vi "MIO Get QCurve Multi.vi"(1 "Lower Limit":sgl format="%.2f", 2 "Upper Limit":sgl format="%.2f", 3 "Num Sweeps":i32=1) -> (0 "Waveform Graph":dbl[](graph))   [LabVIEW 2009]
uses:
  <vilib>/Daq/zadvd.llb/AO Buffer Write (scaled array).vi
  QCA Global.vi
  <vilib>/Daq/Ai.llb/AI Read (scaled array).vi
panel:
  in  "Multiplicity":i32=1
  out "Tune":dbl(slide) scale=-1.0..1.0 scale format="%.2f"
  out "Triangle Wave":dbl[](graph)=[-1.0, -0.996, -0.992, -0.988, -0.984, -0.98, -0.976, -0.972, -0.968, -0.964, -0.96, -0.956, -0.952, -0.948, -0.944, -0.94, -0.9359999999999999, -0.9319999999999999, -0.928, -0.924, -0.92, -0.916, -0.912, -0.908, -0.904, -0.9, -0.896, -0.892, -0.888, -0.884, -0.88, -0.876, -0.872, -0.868, -0.864, -0.86, -0.856, -0.852, -0.848, -0.844, -0.84, -0.836, -0.832, -0.8280000000000001, -0.8240000000000001, -0.8200000000000001, -0.8160000000000001, -0.812, -0.808, -0.804, -0.8, -0.796, -0.792, -0.788, -0.784, -0.78, -0.776, -0.772, -0.768, -0.764, -0.76, -0.756, -0.752, -0.748, -0.744, -0.74, -0.736, -0.732, -0.728, -0.724, -0.72, -0.716, -0.712, -0.708, -0.704, -0.7, -0.696, -0.692, -0.688, -0.6839999999999999, -0.6799999999999999, -0.6759999999999999, -0.6719999999999999, -0.6679999999999999, -0.6639999999999999, -0.6599999999999999, -0.656, -0.652, -0.648, -0.644, -0.64, -0.636, -0.632, -0.628, -0.624, -0.62, -0.616, -0.612, -0.608, -0.604, -0.6, -0.596, -0.5920000000000001, -0.5880000000000001, -0.5840000000000001, -0.5800000000000001, -0.5760000000000001, -0.5720000000000001, -0.5680000000000001, -0.5640000000000001, -0.56, -0.556, -0.552, -0.548, -0.544, -0.54, -0.536, -0.532, -0.528, -0.524, -0.52, -0.516, -0.512, -0.508, -0.504, -0.5, -0.496, -0.492, -0.488, -0.484, -0.48, -0.476, -0.472, -0.46799999999999997, -0.46399999999999997, -0.45999999999999996, -0.45599999999999996, -0.45199999999999996, -0.44799999999999995, -0.44399999999999995, -0.43999999999999995, -0.43600000000000005, -0.43200000000000005, -0.42800000000000005, -0.42400000000000004, -0.42000000000000004, -0.41600000000000004, -0.41200000000000003, -0.40800000000000003, -0.404, -0.4, -0.396, -0.392, -0.388, -0.384, -0.38, -0.376, -0.372, -0.368, -0.364, -0.36, -0.356, -0.352, -0.348, -0.344, -0.33999999999999997, -0.33599999999999997, -0.33199999999999996, -0.32799999999999996, -0.32399999999999995, -0.31999999999999995, -0.31599999999999995, -0.31200000000000006, -0.30800000000000005, -0.30400000000000005, -0.30000000000000004, -0.29600000000000004, -0.29200000000000004, -0.28800000000000003, -0.28400000000000003, -0.28, -0.276, -0.272, -0.268, -0.264, -0.26, -0.256, -0.252, -0.248, -0.244, -0.24, -0.236, -0.23199999999999998, -0.22799999999999998, -0.22399999999999998, -0.21999999999999997, -0.21599999999999997, -0.21199999999999997, -0.20799999999999996, -0.20399999999999996, -0.19999999999999996, -0.19599999999999995, -0.19199999999999995, -0.18799999999999994, -0.18400000000000005, -0.18000000000000005, -0.17600000000000005, -0.17200000000000004, -0.16800000000000004, -0.16400000000000003, -0.16000000000000003, -0.15600000000000003, -0.15200000000000002, -0.14800000000000002, -0.14400000000000002, -0.14, -0.136, -0.132, -0.128, -0.124, -0.12, -0.11599999999999999, -0.11199999999999999, -0.10799999999999998, -0.10399999999999998, -0.09999999999999998, -0.09599999999999997, -0.09199999999999997, -0.08799999999999997, -0.08399999999999996, -0.07999999999999996, -0.07599999999999996, -0.07199999999999995, -0.06799999999999995, -0.06399999999999995, -0.06000000000000005, -0.05600000000000005, -0.052000000000000046, -0.04800000000000004, -0.04400000000000004, -0.040000000000000036, -0.03600000000000003, -0.03200000000000003, -0.028000000000000025, -0.02400000000000002, -0.020000000000000018, -0.016000000000000014, -0.01200000000000001, -0.008000000000000007, -0.0040000000000000036, 0.0, 0.0040000000000000036, 0.008000000000000007, 0.01200000000000001, 0.016000000000000014, 0.020000000000000018, 0.02400000000000002, 0.028000000000000025, 0.03200000000000003, 0.03600000000000003, 0.040000000000000036, 0.04400000000000004, 0.04800000000000004, 0.052000000000000046, 0.05600000000000005, 0.06000000000000005, 0.06400000000000006, 0.06800000000000006, 0.07200000000000006, 0.07600000000000007, 0.08000000000000007, 0.08400000000000007, 0.08800000000000008, 0.09200000000000008, 0.09600000000000009, 0.10000000000000009, 0.10400000000000009, 0.1080000000000001, 0.1120000000000001, 0.1160000000000001, 0.1200000000000001, 0.12400000000000011, 0.1279999999999999, 0.1319999999999999, 0.1359999999999999, 0.1399999999999999, 0.1439999999999999, 0.1479999999999999, 0.1519999999999999, 0.15599999999999992, 0.15999999999999992, 0.16399999999999992, 0.16799999999999993, 0.17199999999999993, 0.17599999999999993, 0.17999999999999994, 0.18399999999999994, 0.18799999999999994, 0.19199999999999995, 0.19599999999999995, 0.19999999999999996, 0.20399999999999996, 0.20799999999999996, 0.21199999999999997, 0.21599999999999997, 0.21999999999999997, 0.22399999999999998, 0.22799999999999998, 0.23199999999999998, 0.236, 0.24, 0.244, 0.248, 0.252, 0.256, 0.26, 0.264, 0.268, 0.272, 0.276, 0.28, 0.28400000000000003, 0.28800000000000003, 0.29200000000000004, 0.29600000000000004, 0.30000000000000004, 0.30400000000000005, 0.30800000000000005, 0.31200000000000006, 0.31600000000000006, 0.32000000000000006, 0.32400000000000007, 0.32800000000000007, 0.3320000000000001, 0.3360000000000001, 0.3400000000000001, 0.3440000000000001, 0.3480000000000001, 0.3520000000000001, 0.3560000000000001, 0.3600000000000001, 0.3640000000000001, 0.3680000000000001, 0.3720000000000001, 0.3759999999999999, 0.3799999999999999, 0.3839999999999999, 0.3879999999999999, 0.3919999999999999, 0.3959999999999999, 0.3999999999999999, 0.4039999999999999, 0.4079999999999999, 0.4119999999999999, 0.4159999999999999, 0.41999999999999993, 0.42399999999999993, 0.42799999999999994, 0.43199999999999994, 0.43599999999999994, 0.43999999999999995, 0.44399999999999995, 0.44799999999999995, 0.45199999999999996, 0.45599999999999996, 0.45999999999999996, 0.46399999999999997, 0.46799999999999997, 0.472, 0.476, 0.48, 0.484, 0.488, 0.492, 0.496, 0.5, 0.504, 0.508, 0.512, 0.516, 0.52, 0.524, 0.528, 0.532, 0.536, 0.54, 0.544, 0.548, 0.552, 0.556, 0.56, 0.5640000000000001, 0.5680000000000001, 0.5720000000000001, 0.5760000000000001, 0.5800000000000001, 0.5840000000000001, 0.5880000000000001, 0.5920000000000001, 0.5960000000000001, 0.6000000000000001, 0.6040000000000001, 0.6080000000000001, 0.6120000000000001, 0.6160000000000001, 0.6200000000000001, 0.6240000000000001, 0.6279999999999999, 0.6319999999999999, 0.6359999999999999, 0.6399999999999999, 0.6439999999999999, 0.6479999999999999, 0.6519999999999999, 0.6559999999999999, 0.6599999999999999, 0.6639999999999999, 0.6679999999999999, 0.6719999999999999, 0.6759999999999999, 0.6799999999999999, 0.6839999999999999, 0.688, 0.692, 0.696, 0.7, 0.704, 0.708, 0.712, 0.716, 0.72, 0.724, 0.728, 0.732, 0.736, 0.74, 0.744, 0.748, 0.752, 0.756, 0.76, 0.764, 0.768, 0.772, 0.776, 0.78, 0.784, 0.788, 0.792, 0.796, 0.8, 0.804, 0.808, 0.812, 0.8160000000000001, 0.8200000000000001, 0.8240000000000001, 0.8280000000000001, 0.8320000000000001, 0.8360000000000001, 0.8400000000000001, 0.8440000000000001, 0.8480000000000001, 0.8520000000000001, 0.8560000000000001, 0.8600000000000001, 0.8640000000000001, 0.8680000000000001, 0.8720000000000001, 0.8759999999999999, 0.8799999999999999, 0.8839999999999999, 0.8879999999999999, 0.8919999999999999, 0.8959999999999999, 0.8999999999999999, 0.9039999999999999, 0.9079999999999999, 0.9119999999999999, 0.9159999999999999, 0.9199999999999999, 0.9239999999999999, 0.9279999999999999, 0.9319999999999999, 0.9359999999999999, 0.94, 0.944, 0.948, 0.952, 0.956, 0.96, 0.964, 0.968, 0.972, 0.976, 0.98, 0.984, 0.988, 0.992, 0.996]
  # "A\nD\nD\n\nP\nH\nA\nS\nE"
  # "R\nE\nM\nO\nV\nE\n\nP\nH\nA\nS\nE"
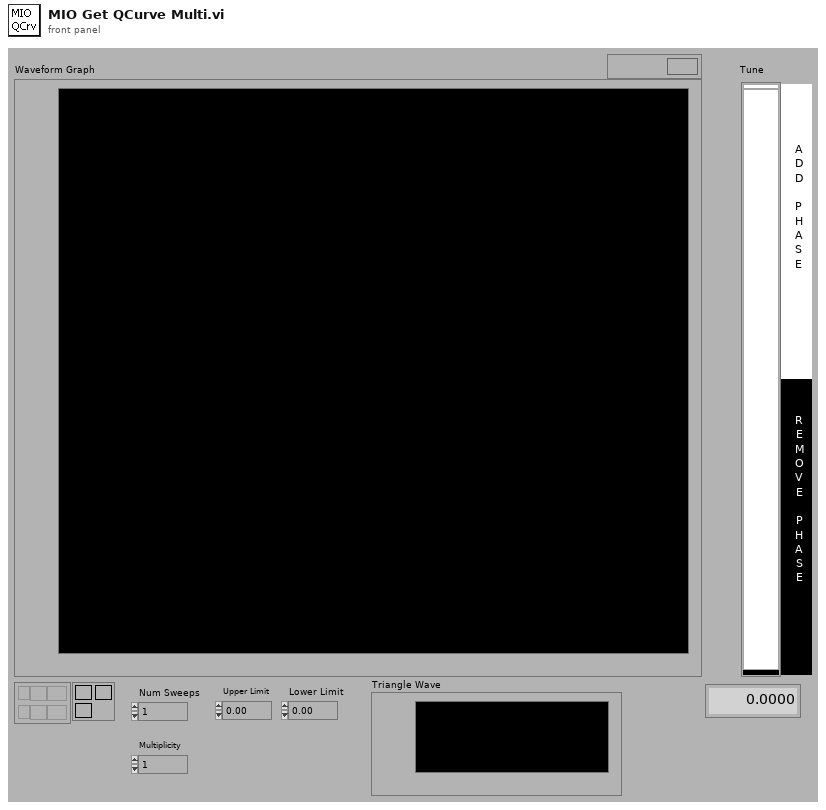
[diagram p1: front panel]
types:
  T1 = cluster{"upper limit (V)":sgl, "lower limit (V)":sgl, "reference source":enum16{"no change", "internal", "external"}}[]
  T2 = enum16{"ungated/software start", "count while high", "count while low", "start on rising edge", "start on falling edge", "restart on each rising edge", "restart on each falling edge"}
  T3 = enum16{"no change", "none", "trigger on rising edge", "trigger on falling edge", "pause while gate is TTL high", "pause while gate is TTL low"}
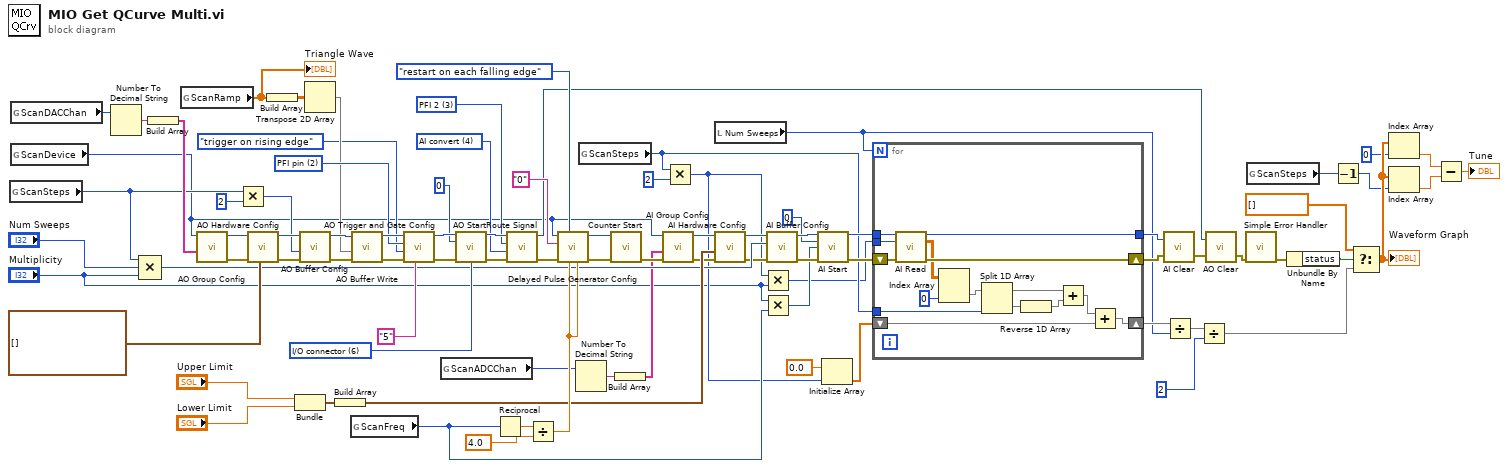
[diagram p0: block diagram]
diagram:
  w67 = u16 4 items=["no change", "none", "AI start trigger", "AI stop trigger", "AI convert", "GPCTR 1 source", "GPCTR 1 gate", "AO update", "AO start trigger", "AI scan start", "GPCTR  0 source", "GPCTR  0 gate", "GPCTR  0 output", "RTSI 0", "RTSI 1", "RTSI 2", "RTSI 3", "RTSI 4", "RTSI 5", "RTSI 6", "RTSI clock", "board clock", "PLL input pin", "marker out", "SYNC out", "analog trigger circuit output", "end of acquisition", "frequency output", "high", "low", "SCANCLK", "inverted voltmeter complete", "voltmeter complete", "GPCTR n source", "GPCTR n gate", "GPCTR n output", "PFI n", "AI scan in progress", "(Reserved_1)", "(Reserved_2)", "stable 10MHz"] ("signal source")
  w68 = u16 3 items=["no change", "PFI 0", "PFI 1", "PFI 2", "PFI 3", "PFI 4", "PFI 5", "PFI 6", "PFI 7", "PFI 8", "PFI 9", "GPCTR 0 output", "RTSI 0", "RTSI 1", "RTSI 2", "RTSI 3", "RTSI 4", "RTSI 5", "RTSI 6", "RTSI clock", "board clock", "PLL reference clock", "SCANCLK", "I/O connector", "PFI n", "start trigger", "configurable filter", "PXI backplane clock"] ("signal name")
  w69 = u16 6 items=["no change", "internal", "counter 1", "counter 2", "counter 3", "counter 5", "I/O connector", "RTSI connection", "PFI pin, low to high", "PFI pin, high to low", "RTSI pin, low to high", "RTSI pin, high to low", "GPCTR 1 output, low to high", "GPCTR 1 output, high to low", "ATCOUT, low to high", "ACTOUT, high to low", "internal clock 2"] ("clock source (internal:1)")
  w71 = u16 2 items=["no change", "none", "PFI pin", "RTSI pin", "AI start trigger", "ATCOUT", "trigger input connector"] ("trigger or gate source (0: no change)")
  n1 = global read "QCA Global.vi" "ScanSteps"() -> (w10:i32)
  n2 = global read "QCA Global.vi" "ScanDACChan"() -> (w11:i32)
  n3 = global read "QCA Global.vi" "ScanDevice"() -> (w9:i32)
  n4 = Number To Decimal String(number=w11) -> (decimal integer string=w28:string)  [unwired: 1 in]
  n5 = Compound Arithmetic op=MULTIPLY(w10, "Num Sweeps", "Multiplicity") -> (w45:i32)
  n6 = Build Array(w28) -> (w27:string[])
  n7 = global read "QCA Global.vi" "ScanRamp"() -> (w32:dbl[])
  "Triangle Wave" <- w32
  n8 = call <vilib>:"AO Group Config.vi"("channel list (empty)"=w27, "device"=w9) -> ("error out"=w63:errorcluster, "task ID out"=w78:u32)  [unwired: 7 in, 1 out]
  n9 = Multiply(x=w10, y=2) -> (x*y=w54:i32)
  n10 = call <vilib>:"AO Hardware Config.vi"("limit settings (no change)"=T1 [], "error in (no error)"=w63, "task ID"=w78) -> ("error out"=w86:errorcluster, "task ID out"=w77:u32)  [unwired: 6 in, 1 out]
  n11 = Build Array(w32) -> (w57:dbl[][])
  n12 = Bundle("Upper Limit"="Upper Limit", "Lower Limit"="Lower Limit") -> (w53:cluster{"Upper Limit":sgl, "Lower Limit":sgl})  [unwired: 1 in]
  n13 = call <vilib>:"AO Buffer Config.vi"("error in (no error)"=w86, "number of updates\n (-1: no change)"=w54, "task ID"=w77) -> ("error out"=w61:errorcluster, "task ID out"=w76:u32)  [unwired: 7 in]
  n14 = Transpose 2D Array(2D array=w57) -> (transposed array=w56:dbl[][])
  n15 = Build Array(w53) -> (w49:cluster{"Upper Limit":sgl, "Lower Limit":sgl}[])
  n16 = global read "QCA Global.vi" "ScanFreq"() -> (w5:i32)
  n17 = call-poly <vilib>:"AO Buffer Write.vi"("error in (no error)"=w61, "scaled data (empty)"=w56, "task ID"=w76) -> ("error out"=w62:errorcluster, "task ID out"=w75:u32)  [unwired: 6 in, 1 out]
  n18 = call <vilib>:"AO Trigger and Gate Config.vi"("trigger or gate  source specification"="5", "error in (no error)"=w62, "trigger or gate condition (0: no change)"=T3."trigger on rising edge", "trigger or gate source (0: no change)"=w71, "task ID"=w75) -> ("error out"=w80:errorcluster, "task ID out"=w74:u32)  [unwired: 5 in]
  n19 = global read "QCA Global.vi" "ScanADCChan"() -> (w8:i32)
  n20 = call <vilib>:"AO Start.vi"("taskID in"=w74, "number of buffer iterations (1)"=0, "error in (no error)"=w80, "clock source (internal:1)"=w69) -> ("taskID out"=w72:u32, "error out"=w85:errorcluster)  [unwired: 9 in, 1 out]
  n21 = Reciprocal(x=w5) -> (1/x=w59:dbl)
  n22 = call <vilib>:"Route Signal.vi"("error in (no error)"=w85, "signal source"=w67, "signal name"=w68, "task ID"=w72) -> ("error out"=w84:errorcluster, "task ID out"=w64:u32)  [unwired: 6 in]
  n23 = Divide(x=w59, y=sgl 4.0 ("Input")) -> (x/y=w60:dbl)
  n24 = call <vilib>:"Delayed Pulse Generator Config.vi"("pulse width (s or cycles)"=w60, "pulse delay (s or cycles)"=w60, "gate mode (ungated:0)"=T2."restart on each falling edge", "error in (no error)"=w84, "counter"="0", "device"=w9) -> ("error out"=w83:errorcluster, "taskID"=w73:u32)  [unwired: 2 in, 2 out]
  n25 = Number To Decimal String(number=w8) -> (decimal integer string=w30:string)  [unwired: 1 in]
  n26 = global read "QCA Global.vi" "ScanSteps"() -> (w6:i32)
  n27 = call <vilib>:"Counter Start.vi"("error in (no error)"=w83, "taskID"=w73) -> ("error out"=w82:errorcluster)  [unwired: 8 in, 1 out]
  n28 = Build Array(w30) -> (w29:string[])
  n29 = call <vilib>:"AI Group Config.vi"("error in (no error)"=w82, "channel scan list (empty)"=w29, "device"=w9) -> ("error out"=w42:errorcluster, "task ID"=w41:u32)  [unwired: 6 in, 1 out]
  n30 = Multiply(x=w6, y=2) -> (x*y=w3:i32)
  n31 = local read "Num Sweeps"() -> (w22:i32)
  n32 = call <vilib>:"AI Hardware Config.vi"("error in (no error)"=w42, "input limits(no change)"=w49, "task ID"=w41) -> ("error out"=w44:errorcluster, "task ID out"=w40:u32)  [unwired: 6 in, 1 out]
  n33 = Multiply(x=w3, y="Multiplicity") -> (x*y=w1:i32)
  n34 = Multiply(x="Multiplicity", y=w5) -> (x*y=w4:i32)
  n35 = call <vilib>:"AI Buffer Config.vi"("error in (no error)"=w44, "scans per buffer (-1: no change)"=w45, "task ID"=w40) -> ("error out"=w43:errorcluster, "task ID out"=w39:u32)  [unwired: 7 in]
  n36 = call <vilib>:"AI Start.vi"("taskID in"=w39, "number of scans to acquire (-1)"=0, "scan rate (1000 scans/sec)"=w4, "error in (no error)"=w43) -> ("taskID out"=w34:u32, "error out"=w33:errorcluster)  [unwired: 8 in, 2 out]
  n37 = Initialize Array(sgl 0.0 ("Element Data"), w3) -> (w36:sgl[])
  n38 = for {
    N: w22 -> [_]
    tunnel: w1 -> [w101]
    shift-right: [w99] -> w46
    shift-left: w33 -> [w100]
    tunnel: w34 -> [w98]
    tunnel: [w97] -> w47
    tunnel: w6 -> [w91]
    shift-right: [w89] -> w23
    shift-left: w36 -> [w90]
    n39 = call-poly <vilib>:"AI Read.vi"("taskID in"=w98, "number of scans to read (-1:all)"=w101, "error in (no error)"=w100) -> ("taskID out"=w97:u32, "scaled data"=w92:sgl[][], "error out"=w99:errorcluster)  [unwired: 7 in, 3 out]
    n40 = Index Array(array=w92, index (col)=0 ("Index")) -> (element=w88:sgl[])  [unwired: 1 in]
    n41 = Split 1D Array(array=w88, index=w91) -> (first subarray=w96:sgl[], second subarray=w94:sgl[])
    n42 = Reverse 1D Array(array=w94) -> (reversed array=w95:sgl[])
    n43 = Add(x=w96, y=w95) -> (x+y=w87:sgl[])
    n44 = Add(x=w87, y=w90) -> (x+y=w89:sgl[])
  }
  n45 = call <vilib>:"AI Clear.vi"("error in (no error)"=w46, "taskID in"=w47) -> ("error out"=w48:errorcluster)  [unwired: 4 in, 1 out]
  n46 = Divide(x=w23, y=w22) -> (x/y=w21:sgl[])
  n47 = Divide(x=w21, y=2) -> (x/y=w19:sgl[])
  n48 = call <vilib>:"AO Clear.vi"("error in (no error)"=w48, "taskID in"=w64) -> ("error out"=w81:errorcluster)  [unwired: 4 in, 1 out]
  n49 = call <vilib>:"Simple Error Handler.vi"("error in (no error)"=w81) -> ("error out"=w25:errorcluster)  [unwired: 4 in, 4 out]
  n50 = global read "QCA Global.vi" "ScanSteps"() -> (w7:i32)
  n51 = Unbundle By Name(w25) -> ("status"=w24:bool)
  n52 = Decrement(x=w7) -> (x-1=w13:i32)
  n53 = Select(t=dbl[] [], s=w24, f=w19) -> (s? t:f=w15:dbl[])
  "Waveform Graph" <- w15
  n54 = Index Array(array=w15, index=0 ("Index")) -> (element=w16:dbl)
  n55 = Index Array(array=w15, index=w13) -> (element=w17:dbl)
  n56 = Subtract(x=w16, y=w17) -> (x-y=→"Tune":dbl)
